vi "SEN_Loop.vi"() -> ()   [LabVIEW 2020, in "Template_SEN.lvlib"]
uses:
  Template_SEN.lvlib
  ENUM_SEN_State.ctl
  ENUM_SEN_Action.ctl
  Utility/Global_STOP.vi
  Global_CMD_SEN_Data In.vi
  Global_SEN_Data Out.vi
panel:
  out "Input Bool Data":bool
  out "Output DBL Data":dbl
  out "Cycle Time (S)":dbl format="%.3g"
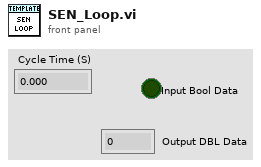
[diagram p1: front panel]
types:
  T1 = typedef "Template_SEN.lvlib/ENUM_SEN_State.ctl" = enum16{"Startup", "Reset", "Enable", "Disable", "Shutdown"}
  T2 = typedef "Template_SEN.lvlib/ENUM_SEN_Action.ctl" = enum16{"No Action", "Reset Time", "Reset Enable", "Reset Disable", "Read Enable", "Read Disable"}
  T3 = cluster{"Sensor Ref 0":cluster{i32}, "State":T1, "Previous State":T1, "Current Time":timestamp, "Previous Time":timestamp, "Start Time":timestamp, "Target Time (ms)":u32, "Cycle Time(S)":dbl, "SEN Input":bool, "SEN Output DBL":dbl, "Read Enable":bool}
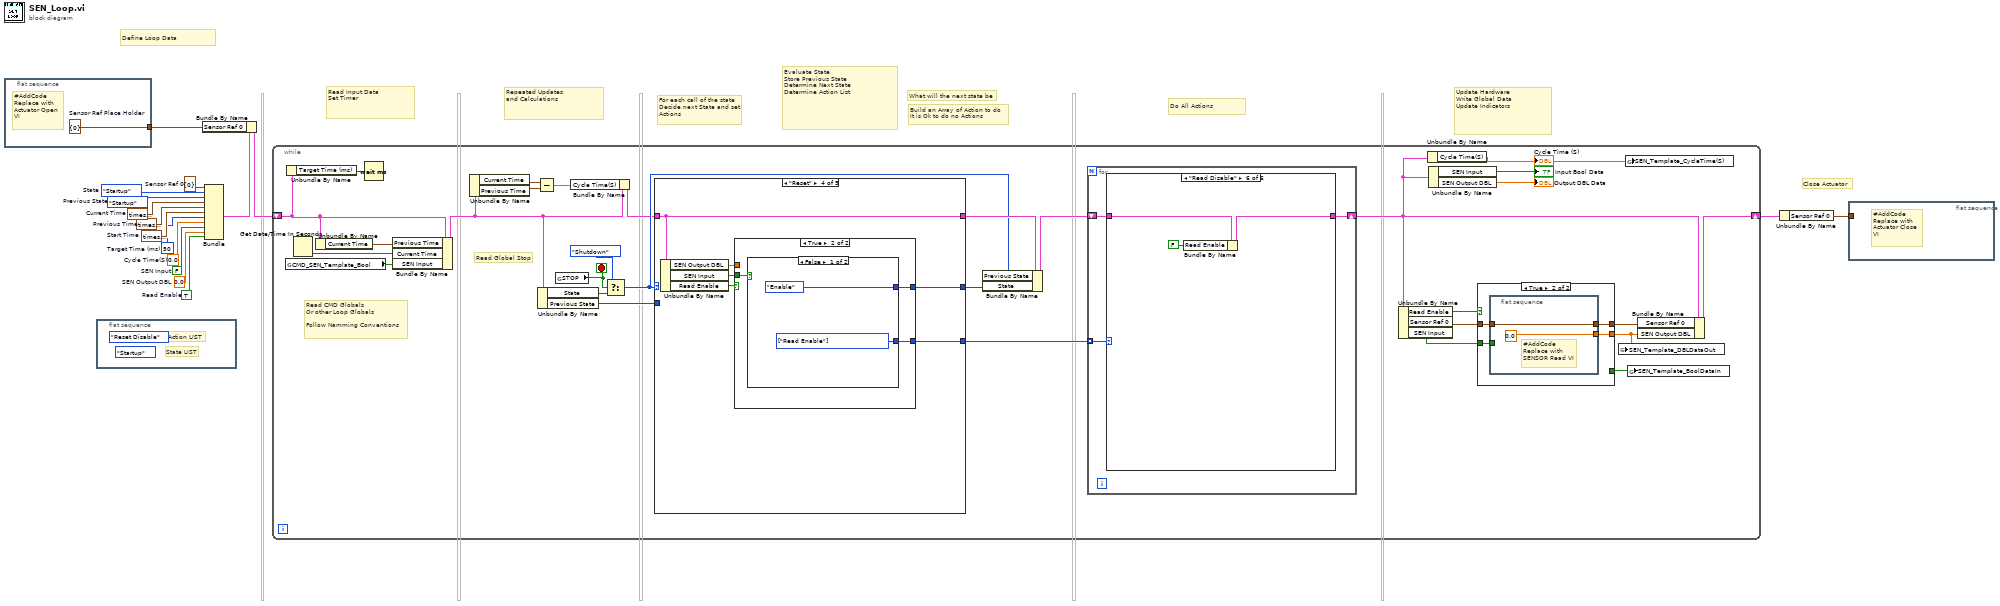
[diagram p0: block diagram]
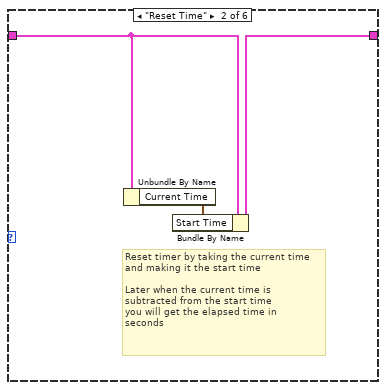
[diagram p4: hidden frame]
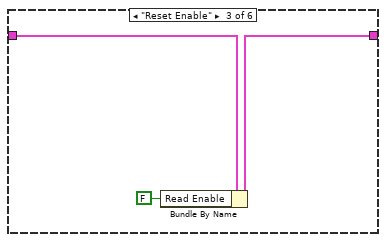
[diagram p5: hidden frame]
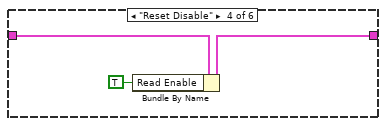
[diagram p6: hidden frame]
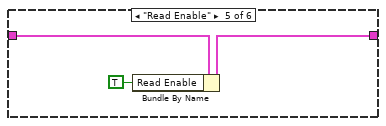
[diagram p7: hidden frame]
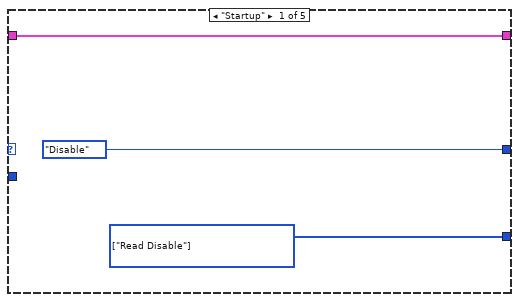
[diagram p8: hidden frame]
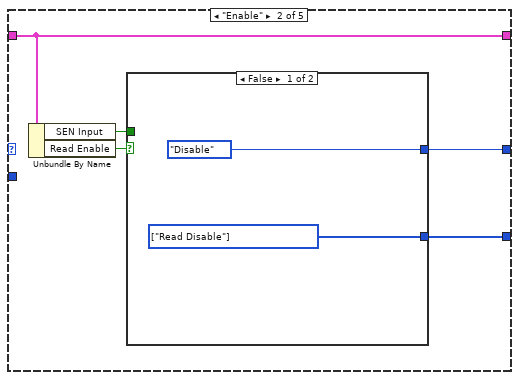
[diagram p9: hidden frame]
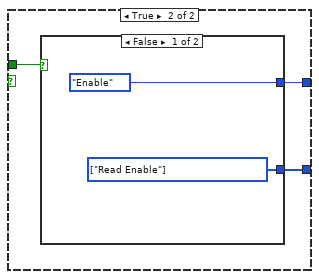
[diagram p10: hidden frame]
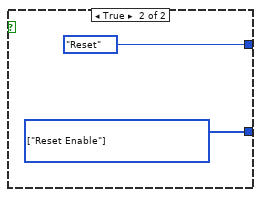
[diagram p11: hidden frame]
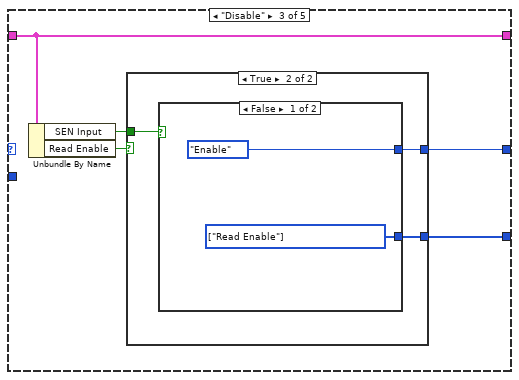
[diagram p12: hidden frame]
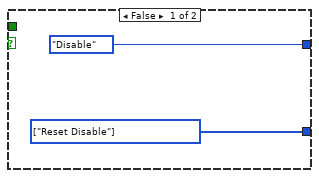
[diagram p13: hidden frame]
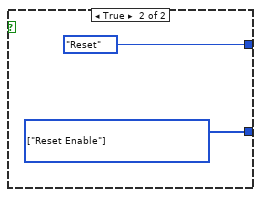
[diagram p14: hidden frame]
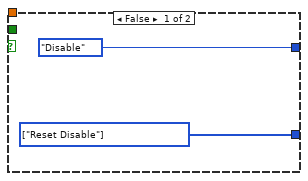
[diagram p15: hidden frame]
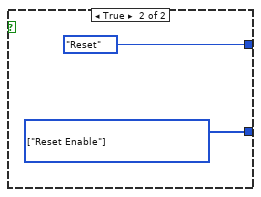
[diagram p16: hidden frame]
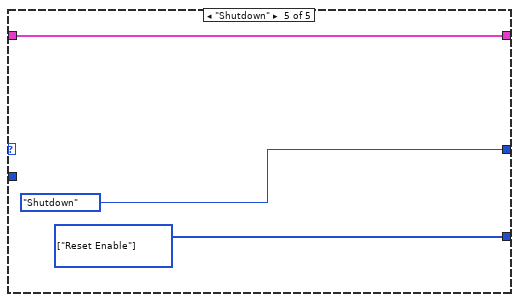
[diagram p17: hidden frame]
diagram:
  w4 = cluster{i32} {0}  # Sensor Ref 0
  w5 = TRUE  # Read Enable
  w8 = 0.0  # Cycle Time(S)
  w9 = ENUM_SEN_State."Startup"  # Previous State
  w10 = timestamp(0 s since 1904-01-01)  # Previous Time
  w11 = u32 50  # Target Time (ms)
  w12 = 0.0  # SEN Output DBL
  w13 = FALSE  # SEN Input
  w14 = timestamp(0 s since 1904-01-01)  # Start Time
  w15 = timestamp(0 s since 1904-01-01)  # Current Time
  w16 = ENUM_SEN_State."Startup"  # State
  # "Build an Array of Action to do\nIt is Ok to do no Actions"
  # "What will the next state be"
  # "For each call of the state\nDecide next State and set\nActions"
  # "Close Actuator"
  # "Define Loop Data"
  # "Repeated Updates\nand Calculations"
  # "Read Input Data\nSet Timer"
  # "Evaluate State\nStore Previous State\nDetermine Next State\nDetermine Action List"
  # "Do All Actions"
  # "Update Hardware\nWrite Global Data\nUpdate Indicators"
  n1 = flat-sequence {
    tunnel: [w17] -> w1
    frame #0 {
      w17 = cluster{i32} {0}  # Sensor Ref Place Holder
      # "#AddCode\nReplace with \nActuator Open\nVI"
    }
  }
  n2 = flat-sequence {
    frame #0 {
      (unwired) ENUM_SEN_State."Startup" ("State")
      (unwired) ENUM_SEN_Action."Reset Disable" ("Action")
      # "State LIST"
      # "Action LIST"
    }
  }
  n3 = Bundle("Sensor Ref 0"=w4, "State"=w16, "Previous State"=w9, "Current Time"=w15, "Previous Time"=w10, "Start Time"=w14, "Target Time (ms)"=w11, "Cycle Time(S)"=w8, "SEN Input"=w13, "SEN Output DBL"=w12, "Read Enable"=w5) -> (w3:T3)  [unwired: 1 in]
  n4 = Bundle By Name(cluster=w3, "Sensor Ref 0"=w1) -> (w2:T3)
  n5 = while {
    shift-right: [w23] -> w6
    shift-left: w2 -> [w38]
    stop <- w43 stop-if-true
    # "Read CMD Globals\nOr other Loop Globals\n\nFollow Namming Conventions"
    # "Read Global Stop"
    n6 = global read "Global_CMD_SEN_Data In.vi" "CMD_SEN_Template_Bool"() -> (w27:bool)
    n7 = Unbundle By Name(w38) -> ("Target Time (ms)"=w40:u32)
    n8 = Get Date/Time In Seconds() -> (seconds since 1Jan1904=w47:timestamp)
    n9 = Unbundle By Name(w38) -> ("Current Time"=w39:timestamp)
    n10 = Wait (ms)(milliseconds to wait=w40) -> ()  [unwired: 1 out]
    n11 = Bundle By Name(cluster=w38, "Previous Time"=w39, "Current Time"=w47, "SEN Input"=w27) -> (w32:T3)
    n12 = Unbundle By Name(w32) -> ("Current Time"=w33:timestamp, "Previous Time"=w34:timestamp)
    n13 = Subtract(x=w33, y=w34) -> (x-y=w30:dbl)
    n14 = Unbundle By Name(w32) -> ("State"=w41:T1, "Previous State"=w37:T1)
    n15 = global read "Global_STOP.vi" "STOP"() -> (w43:bool)
    n16 = Bundle By Name(cluster=w32, "Cycle Time(S)"=w30) -> (w31:T3)
    n17 = Select(t=ENUM_SEN_State."Shutdown" ("State"), s=w43, f=w41) -> (s? t:f=w35:T1)
    n18 = case shown="\"Reset\"" w35 {
      tunnel: w31 -> [w77 w80 w94 w109 w123]
      tunnel: [w77 w80 w94 w109 w123] -> w45
      tunnel: [ENUM_SEN_State."Disable" ("State") w81 w95 w110 ENUM_SEN_State."Shutdown" ("State")] -> w44
      tunnel: [w76 w82 w96 w111 w121] -> w29
      tunnel: w37 -> [_ _ _ _ _]
      frame "Startup" {
        w76 = T2[] [enum."Read Disable"] items=["No Action", "Reset Time", "Reset Enable", "Reset Disable", "Read Enable", "Read Disable"] ("Actions")
      }
      frame "Enable" {
        n19 = Unbundle By Name(w80) -> ("SEN Input"=w78:bool, "Read Enable"=w79:bool)
        n20 = case shown="False" w79 {
          tunnel: [w83 w87] -> w82
          tunnel: [ENUM_SEN_State."Disable" ("State") w86] -> w81
          tunnel: w78 -> [_ w85]
          frame False {
            w83 = T2[] [enum."Read Disable"] items=["No Action", "Reset Time", "Reset Enable", "Reset Disable", "Read Enable", "Read Disable"] ("Actions")
          }
          frame True {
            n21 = case shown="False" w85 {
              tunnel: [w88 w91] -> w87
              tunnel: [ENUM_SEN_State."Enable" ("State") ENUM_SEN_State."Reset" ("State")] -> w86
              frame False {
                w88 = T2[] [enum."Read Enable"] items=["No Action", "Reset Time", "Reset Enable", "Reset Disable", "Read Enable", "Read Disable"] ("Actions")
              }
              frame True {
                w91 = T2[] [enum."Reset Enable"] items=["No Action", "Reset Time", "Reset Enable", "Reset Disable", "Read Enable", "Read Disable"] ("Actions")
              }
            }
          }
        }
      }
      frame "Disable" {
        n22 = Unbundle By Name(w94) -> ("SEN Input"=w92:bool, "Read Enable"=w93:bool)
        n23 = case shown="True" w93 {
          tunnel: [w97 w101] -> w96
          tunnel: [ENUM_SEN_State."Disable" ("State") w100] -> w95
          tunnel: w92 -> [_ w99]
          frame False {
            w97 = T2[] [enum."Reset Disable"] items=["No Action", "Reset Time", "Reset Enable", "Reset Disable", "Read Enable", "Read Disable"] ("Actions")
          }
          frame True {
            n24 = case shown="False" w99 {
              tunnel: [w102 w105] -> w101
              tunnel: [ENUM_SEN_State."Enable" ("State") ENUM_SEN_State."Reset" ("State")] -> w100
              frame False {
                w102 = T2[] [enum."Read Enable"] items=["No Action", "Reset Time", "Reset Enable", "Reset Disable", "Read Enable", "Read Disable"] ("Actions")
              }
              frame True {
                w105 = T2[] [enum."Reset Enable"] items=["No Action", "Reset Time", "Reset Enable", "Reset Disable", "Read Enable", "Read Disable"] ("Actions")
              }
            }
          }
        }
      }
      frame "Reset" {
        n25 = Unbundle By Name(w109) -> ("SEN Output DBL"=w106:dbl, "SEN Input"=w107:bool, "Read Enable"=w108:bool)
        n26 = case shown="True" w108 {
          tunnel: [w112 w116] -> w111
          tunnel: [ENUM_SEN_State."Disable" ("State") w115] -> w110
          tunnel: w107 -> [_ w114]
          tunnel: w106 -> [_ _]
          frame False {
            w112 = T2[] [enum."Reset Disable"] items=["No Action", "Reset Time", "Reset Enable", "Reset Disable", "Read Enable", "Read Disable"] ("Actions")
          }
          frame True {
            n27 = case shown="False" w114 {
              tunnel: [w117 w120] -> w116
              tunnel: [ENUM_SEN_State."Enable" ("State") ENUM_SEN_State."Reset" ("State")] -> w115
              frame False {
                w117 = T2[] [enum."Read Enable"] items=["No Action", "Reset Time", "Reset Enable", "Reset Disable", "Read Enable", "Read Disable"] ("Actions")
              }
              frame True {
                w120 = T2[] [enum."Reset Enable"] items=["No Action", "Reset Time", "Reset Enable", "Reset Disable", "Read Enable", "Read Disable"] ("Actions")
              }
            }
          }
        }
      }
      frame "Shutdown" {
        w121 = T2[] [enum."Reset Enable"] items=["No Action", "Reset Time", "Reset Enable", "Reset Disable", "Read Enable", "Read Disable"] ("Actions")
      }
    }
    n28 = Bundle By Name(cluster=w45, "Previous State"=w35, "State"=w44) -> (w46:T3)
    n29 = for {
      tunnel: w29 -> [w58] mode=indexing
      shift-right: [w57] -> w24
      shift-left: w46 -> [w56]
      n30 = case shown="\"Read Disable\"" w58 {
        tunnel: w56 -> [w59 w62 w65 w68 w71 w74]
        tunnel: [w59 w61 w64 w67 w70 w73] -> w57
        frame "No Action" {
        }
        frame "Reset Time" {
          # "Reset timer by taking the current time\nand making it the start time\n\nLater when the current time is \nsubtracted from the start time\nyou will get the elapsed time in \nseconds"
          n31 = Unbundle By Name(w62) -> ("Current Time"=w60:timestamp)
          n32 = Bundle By Name(cluster=w62, "Start Time"=w60) -> (w61:T3)
        }
        frame "Reset Enable" {
          n33 = Bundle By Name(cluster=w65, "Read Enable"=FALSE) -> (w64:T3)
        }
        frame "Reset Disable" {
          n34 = Bundle By Name(cluster=w68, "Read Enable"=TRUE) -> (w67:T3)
        }
        frame "Read Enable" {
          n35 = Bundle By Name(cluster=w71, "Read Enable"=TRUE) -> (w70:T3)
        }
        frame "Read Disable" {
          n36 = Bundle By Name(cluster=w74, "Read Enable"=FALSE) -> (w73:T3)
        }
      }
    }
    n37 = Unbundle By Name(w24) -> ("Read Enable"=w20:bool, "Sensor Ref 0"=w26:cluster{i32}, "SEN Input"=w19:bool)
    n38 = Unbundle By Name(w24) -> ("Cycle Time(S)"=w22:dbl)
    "Cycle Time (S)" <- w22
    n39 = Unbundle By Name(w24) -> ("SEN Input"=→"Input Bool Data":bool, "SEN Output DBL"=→"Output DBL Data":dbl)
    n40 = case shown="True" w20 {
      tunnel: w26 -> [w49 w53]
      tunnel: [w49 w52] -> w25
      tunnel: [_ w51] -> w21
      tunnel: w19 -> [w48 w50]
      tunnel: [w48 _] -> w18
      frame False {
      }
      frame True {
        n41 = flat-sequence {
          tunnel: w53 -> [w55]
          tunnel: [w55] -> w52
          tunnel: [0.0 ("ACT_Template_DBLDataOut")] -> w51
          tunnel: w50 -> [_]
          frame #0 {
            # "#AddCode\nReplace with\nSENSOR Read VI"
          }
        }
      }
    }
    n42 = global write "Global_SEN_Data Out.vi" "SEN_Template_DBLDataOut"(w21) -> ()
    n43 = global write "Global_SEN_Data Out.vi" "SEN_Template_CycleTime(S)"(w22) -> ()
    n44 = global write "Global_SEN_Data Out.vi" "SEN_Template_BoolDataIn"(w18) -> ()
    n45 = Bundle By Name(cluster=w24, "Sensor Ref 0"=w25, "SEN Output DBL"=w21) -> (w23:T3)
  }
  n46 = Unbundle By Name(w6) -> ("Sensor Ref 0"=w7:cluster{i32})
  n47 = flat-sequence {
    tunnel: w7 -> [_]
    frame #0 {
      # "#AddCode\nReplace with \nActuator Close\nVI"
    }
  }
